vi "VerifyContinuousData.vi"() -> ()   [LabVIEW 2017]
panel:
  out "min value":dbl
  out "index of min value":i32
  out "file containing min index":path
  out "index of max value":i32
  in  "Stream?":bool
  out "file containing max index":path
  out "max value":dbl
  in  "Folder":path
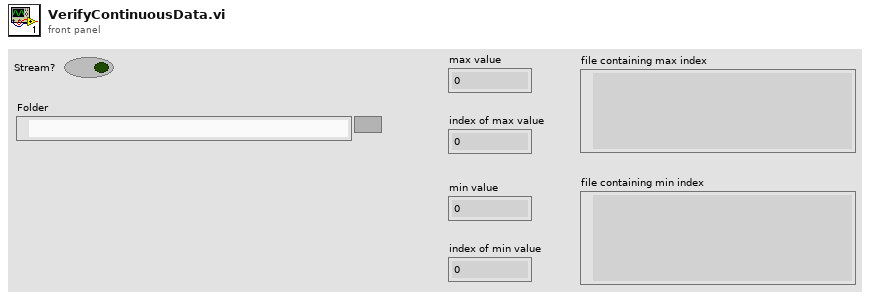
[diagram p1: front panel]
types:
  T1 = enum16{"open", "open or create", "create or replace", "create", "open (read-only)"}
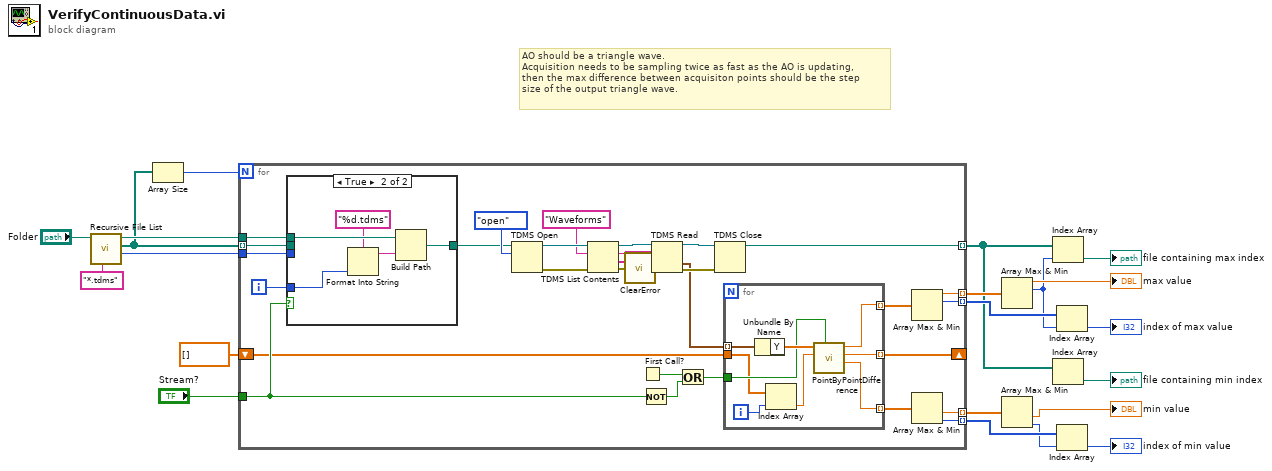
[diagram p0: block diagram]
diagram:
  # "AO should be a triangle wave.\nAcquisition needs to be sampling twice as fast as the AO is updating,\nthen the max difference between acquisiton points should be the step\nsize of the output triangle wave."
  n1 = call <vilib>:"Recursive File List.vi"("pattern"="*.tdms", "Folder Path"="Folder") -> ("Number of Files"=w12:i32, "All Files in Dir"=w13:path[], "dup Folder Path"=w21:path)  [unwired: 5 in, 2 out]
  n2 = Array Size(array=w13) -> (size(s)=w20:i32)
  n3 = for {
    N: w20 -> [_]
    tunnel: w21 -> [w49]
    shift-right: [w38] -> _
    shift-left: dbl[] [] -> [w23]
    tunnel: [w36] -> w19 mode=indexing
    tunnel: [w34] -> w7 mode=indexing
    tunnel: "Stream?" -> [w32]
    tunnel: w13 -> [w30] mode=indexing
    tunnel: w12 -> [w29]
    tunnel: [w28] -> w11 mode=indexing
    tunnel: [w26] -> w8 mode=indexing
    tunnel: [w25] -> w9 mode=indexing
    i -> [w48]
    n4 = case shown="True" w32 {
      tunnel: [w52 w57] -> w50
      tunnel: w49 -> [_ w56]
      tunnel: w48 -> [_ w55]
      tunnel: w30 -> [w52 _]
      tunnel: w29 -> [_ _]
      frame False {
      }
      frame True {
        n5 = Format Into String(format string="%d.tdms", w55) -> (resulting string=w53:string)  [unwired: 2 in, 1 out]
        n6 = Build Path(base path=w56, name or relative path=w53) -> (appended path=w57:path)
      }
    }
    n7 = TDMS Open(10:T1."open" ("operation (0:open)"), 11:w50) -> (0:w46:errorcluster, 3:w47:refnum<k34>)  [unwired: 5 in]
    n8 = TDMS List Contents(4:w46, 6:"Waveforms" ("group name"), 7:w47) -> (0:w22:errorcluster, 1:w42:string[], 2:w43:string, 3:w44:refnum<k34>)
    n9 = call <vilib>:"ClearError.vi"("error in (no error)"=w22) -> ("error out"=w41:errorcluster)
    n10 = First Call?() -> (First Call?: T/F=w33:bool)
    n11 = Not(x=w32) -> (.not. x?=w31:bool)
    n12 = TDMS Read(0:w44, 5:w43, 7:w42, 11:w41) -> (4:w40:refnum<k34>, 10:w37:waveform(dbl)[], 15:w39:errorcluster)  [unwired: 4 in, 3 out]
    n13 = Or(x=w33, y=w31) -> (x .or. y?=w24:bool)
    n14 = TDMS Close(8:w39, 11:w40) -> (3:w34:path)  [unwired: 1 out]
    n15 = for {
      tunnel: w37 -> [w66] mode=indexing
      tunnel: [w64] -> w38 mode=indexing
      tunnel: w23 -> [w59]
      tunnel: [w63] -> w35 mode=indexing
      tunnel: [w62] -> w27 mode=indexing
      tunnel: w24 -> [w61]
      i -> [w60]
      n16 = Unbundle By Name(w66) -> ("Y"=w65:dbl[])
      n17 = Index Array(array=w59, index=w60) -> (element=w58:dbl)
      n18 = call <vilib>:"PointByPointDifference.vi"("reset?"=w61, "initial condition"=w58, "array"=w65) -> ("min difference"=w62:dbl, "last point"=w64:dbl, "max difference"=w63:dbl)  [unwired: 6 in]
    }
    n19 = Array Max & Min(array=w35) -> (max value=w36:dbl, max index (indices)=w28:i32)  [unwired: 2 out]
    n20 = Array Max & Min(array=w27) -> (min value=w26:dbl, min index (indices)=w25:i32)  [unwired: 2 out]
  }
  n21 = Array Max & Min(array=w19) -> (max value=→"max value":dbl, max index (indices)=w6:i32)  [unwired: 2 out]
  n22 = Array Max & Min(array=w8) -> (min value=→"min value":dbl, min index (indices)=w3:i32)  [unwired: 2 out]
  n23 = Index Array(array=w7, index=w6) -> (element=→"file containing max index":path)
  n24 = Index Array(array=w7) -> (element=→"file containing min index":path)  [unwired: 1 in]
  n25 = Index Array(array=w11, index=w6) -> (element=→"index of max value":i32)
  n26 = Index Array(array=w9, index=w3) -> (element=→"index of min value":i32)
